vi "Configure IQ Output.vi"(0 "VISA resource name":refnum<visa-resource-name>, 1 "External Filter (1: Through)":u16(ring)=1 items=["40 MHz", "Through"], 2 "Enable Automatic External Filter (T:Enable)":bool=TRUE, 5 "Modulation Format (1: Dual Modulation)":u16(ring)=1 items=["Custom"=0, "Dual Modulation"=1, "Dual ARB"=2, "Multitone"=3, "Digital Modulation"=4, "Two-tone"=6, "AWGN Real-Time"=7, "AWGN ARB"=8], 7 "I/Q Attenuation Auto Mode (T:Enable)":bool=TRUE, 9 "I/Q Attenuation Level (2 dB)":dbl=2.0, 11 "error in (no error)":errorcluster, 12 "Enable Automatic Modulation Filter (T:Enable)":bool=TRUE, 13 "Modulation Filter (2: Through)":u16(ring)=2 items=["2.1 MHz", "40 MHz", "Through"]) -> (4 "VISA resource name out":refnum<visa-resource-name>, 15 "error out":errorcluster)   [LabVIEW 2018, in "Agilent PSG MXG Series.lvlib"]
doc: "Configures I/Q attenuation, external filter and modulation filter.\n\n<B>Notes:</B>\n(1) This VI is valid only in E8267C, E8257D, E8267D, N5162A, N5182A, N5172B, N5182B.\n\n(2) For E8267C, this VI is valid only when the instrument installs <B>Option 002</B> (Internal baseband generator) or <B>Option 602</B> (Digital bus baseband generator).\n\n(3) For E8267D, this VI is valid only when the instrument installs <B>Option 601</B> or <B>Option 602</B> (Internal baseband generator)."
uses:
  Agilent PSG MXG Series.lvlib
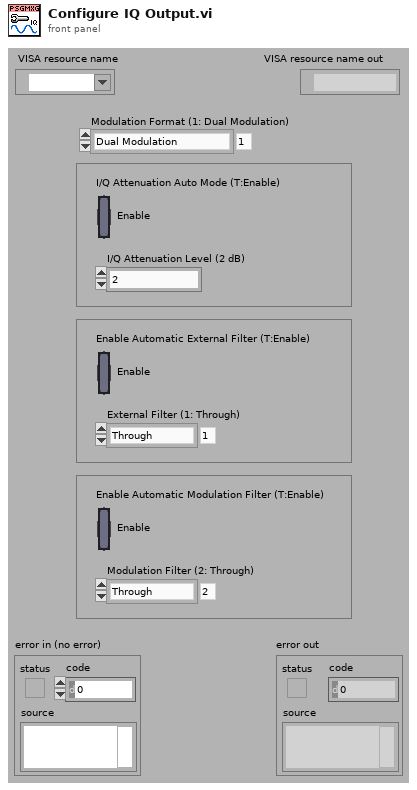
[diagram p1: front panel]
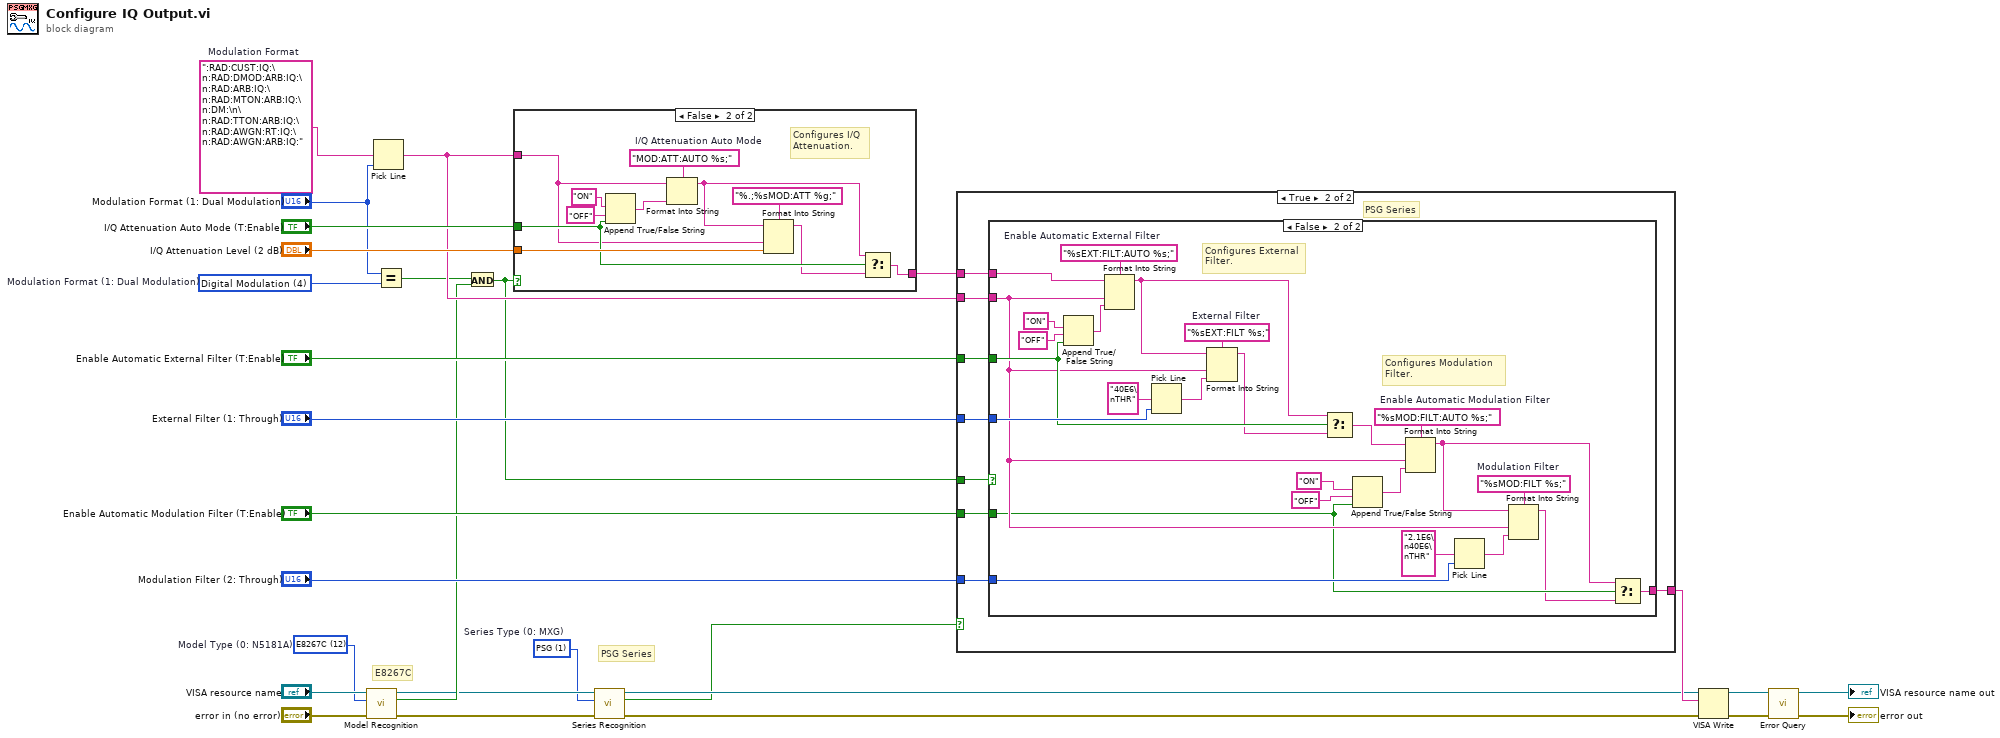
[diagram p0: block diagram]
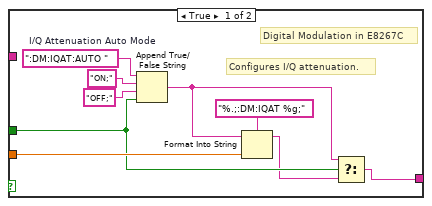
[diagram p2: hidden frame]
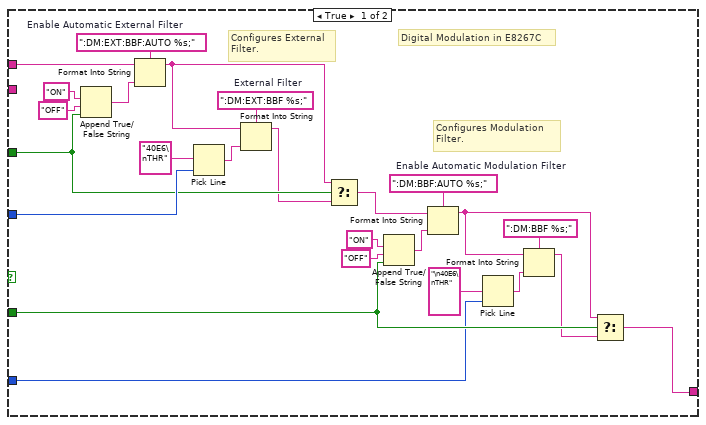
[diagram p4: hidden frame]
diagram:
  w5 = u16 4 items=["Custom"=0, "Dual Modulation"=1, "Dual ARB"=2, "Multitone"=3, "Digital Modulation"=4, "Two-tone"=6, "AWGN Real-Time"=7, "AWGN ARB"=8]  # Modulation Format (1: Dual Modulation)
  w6 = u16 1 items=["MXG-A", "PSG", "PSG-A", "PSG-C", "PSG-D", "MXG-B", "EXG"]  # Series Type (0: MXG)
  w7 = u16 12 items=["N5181A"=0, "N5182A"=1, "N5183A"=2, "N5161A"=3, "N5162A"=4, "E8241A"=5, "E8244A"=6, "E8251A"=7, "E8254A"=8, "E8247C"=10, "E8257C"=11, "E8267C"=12, "E8257D"=15, "E8267D"=16, "N5171B"=17, "N5172B"=18, "N5181B"=19, "N5182B"=20]  # Model Type (0: N5181A)
  w28 = ":RAD:CUST:IQ:\n:RAD:DMOD:ARB:IQ:\n:RAD:ARB:IQ:\n:RAD:MTON:ARB:IQ:\n:DM:\n\n:RAD:TTON:ARB:IQ:\n:RAD:AWGN:RT:IQ:\n:RAD:AWGN:ARB:IQ:"  # Modulation Format
  # "E8267C"
  # "PSG Series"
  n1 = call "Model Recognition.vi"("error in (no error)"="error in (no error)", "Model Type (0: N5181A)"=w7, "VISA resource name"="VISA resource name") -> ("error out"=w13:errorcluster, "Is Model Correct"=w15:bool, "VISA resource name out"=w14:refnum<visa-resource-name>)  [unwired: 6 out]
  n2 = Pick Line(multi-line string=w28, line index="Modulation Format (1: Dual Modulation)") -> (output string=w25:string)  [unwired: 1 out]
  n3 = Equal?(x="Modulation Format (1: Dual Modulation)", y=w5) -> (x = y?=w17:bool)
  n4 = And(x=w17, y=w15) -> (x .and. y?=w12:bool)
  n5 = case shown="False" w12 {
    tunnel: "I/Q Attenuation Level (2 dB)" -> [w34 w43]
    tunnel: "I/Q Attenuation Auto Mode (T:Enable)" -> [w32 w42]
    tunnel: w25 -> [_ w39]
    tunnel: [w29 w38] -> w24
    frame True {
      w37 = ":DM:IQAT:AUTO "  # I/Q Attenuation Auto Mode
      # "Configures I/Q attenuation."
      # "Digital Modulation in E8267C"
      n6 = Append True/False String(1:w32, 2:"OFF;" ("false string"), 3:"ON;" ("true string"), 4:w37) -> (0:w30:string)
      n7 = Format Into String(format string="%.;:DM:IQAT %g;", initial string=w30, w34) -> (resulting string=w31:string)  [unwired: 1 in, 1 out]
      n8 = Select(t=w30, s=w32, f=w31) -> (s? t:f=w29:string)
    }
    frame False {
      w48 = "MOD:ATT:AUTO %s;"  # I/Q Attenuation Auto Mode
      # "Configures I/Q\nAttenuation."
      n9 = Append True/False String(1:w42, 2:"OFF" ("false string"), 3:"ON" ("true string")) -> (0:w47:string)  [unwired: 1 out]
      n10 = Format Into String(format string=w48, initial string=w39, w47) -> (resulting string=w40:string)  [unwired: 1 in, 1 out]
      n11 = Format Into String(format string="%.;%sMOD:ATT %g;", initial string=w40, w39, w43) -> (resulting string=w41:string)  [unwired: 1 in, 1 out]
      n12 = Select(t=w40, s=w42, f=w41) -> (s? t:f=w38:string)
    }
  }
  n13 = call "Series Recognition.vi"("error in (no error)"=w13, "Series Type (0: MXG)"=w6, "VISA resource name"=w14) -> ("error out"=w2:errorcluster, "Is Series Correct"=w1:bool, "VISA resource name out"=w3:refnum<visa-resource-name>)  [unwired: 6 out]
  n14 = case shown="True" w1 {
    tunnel: w25 -> [_ w54]
    tunnel: w24 -> [w49 w57]
    tunnel: "Enable Automatic External Filter (T:Enable)" -> [_ w55]
    tunnel: "External Filter (1: Through)" -> [_ w56]
    tunnel: "Enable Automatic Modulation Filter (T:Enable)" -> [_ w52]
    tunnel: "Modulation Filter (2: Through)" -> [_ w53]
    tunnel: [w49 w51] -> w4
    tunnel: w12 -> [_ w50]
    frame False {
      # "MXG, EXG Series"
    }
    frame True {
      # "PSG Series"
      n15 = case shown="False" w50 {
        tunnel: w57 -> [w82 w107]
        tunnel: w56 -> [w74 w100]
        tunnel: w55 -> [w73 w99]
        tunnel: w54 -> [_ w90]
        tunnel: w53 -> [w61 w87]
        tunnel: w52 -> [w64 w86]
        tunnel: [w58 w83] -> w51
        frame True {
          w69 = ":DM:BBF:AUTO %s;"  # Enable Automatic Modulation Filter
          w77 = ":DM:EXT:BBF %s;"  # External Filter
          w81 = ":DM:EXT:BBF:AUTO %s;"  # Enable Automatic External Filter
          # "Configures Modulation\nFilter."
          # "Configures External\nFilter."
          # "Digital Modulation in E8267C"
          n16 = Append True/False String(1:w73, 2:"OFF" ("false string"), 3:"ON" ("true string")) -> (0:w80:string)  [unwired: 1 out]
          n17 = Format Into String(format string=w81, initial string=w82, w80) -> (resulting string=w71:string)  [unwired: 1 in, 1 out]
          n18 = Pick Line(multi-line string="40E6\nTHR", line index=w74) -> (output string=w76:string)  [unwired: 1 out]
          n19 = Format Into String(format string=w77, initial string=w71, w76) -> (resulting string=w72:string)  [unwired: 1 in, 1 out]
          n20 = Select(t=w71, s=w73, f=w72) -> (s? t:f=w70:string)
          n21 = Append True/False String(1:w64, 2:"OFF" ("false string"), 3:"ON" ("true string")) -> (0:w68:string)  [unwired: 1 out]
          n22 = Format Into String(format string=w69, initial string=w70, w68) -> (resulting string=w59:string)  [unwired: 1 in, 1 out]
          n23 = Pick Line(multi-line string="\n40E6\nTHR", line index=w61) -> (output string=w62:string)  [unwired: 1 out]
          n24 = Format Into String(format string=":DM:BBF %s;", initial string=w59, w62) -> (resulting string=w60:string)  [unwired: 1 in, 1 out]
          n25 = Select(t=w59, s=w64, f=w60) -> (s? t:f=w58:string)
        }
        frame False {
          w91 = "%sMOD:FILT %s;"  # Modulation Filter
          w95 = "%sMOD:FILT:AUTO %s;"  # Enable Automatic Modulation Filter
          w103 = "%sEXT:FILT %s;"  # External Filter
          w108 = "%sEXT:FILT:AUTO %s;"  # Enable Automatic External Filter
          # "Configures Modulation\nFilter."
          # "Configures External\nFilter."
          n26 = Append True/False String(1:w99, 2:"OFF" ("false string"), 3:"ON" ("true string")) -> (0:w104:string)  [unwired: 1 out]
          n27 = Format Into String(format string=w108, initial string=w107, w90, w104) -> (resulting string=w97:string)  [unwired: 1 in, 1 out]
          n28 = Pick Line(multi-line string="40E6\nTHR", line index=w100) -> (output string=w102:string)  [unwired: 1 out]
          n29 = Format Into String(format string=w103, initial string=w97, w90, w102) -> (resulting string=w98:string)  [unwired: 1 in, 1 out]
          n30 = Select(t=w97, s=w99, f=w98) -> (s? t:f=w96:string)
          n31 = Append True/False String(1:w86, 2:"OFF" ("false string"), 3:"ON" ("true string")) -> (0:w94:string)  [unwired: 1 out]
          n32 = Format Into String(format string=w95, initial string=w96, w90, w94) -> (resulting string=w84:string)  [unwired: 1 in, 1 out]
          n33 = Pick Line(multi-line string="2.1E6\n40E6\nTHR", line index=w87) -> (output string=w89:string)  [unwired: 1 out]
          n34 = Format Into String(format string=w91, initial string=w84, w90, w89) -> (resulting string=w85:string)  [unwired: 1 in, 1 out]
          n35 = Select(t=w84, s=w86, f=w85) -> (s? t:f=w83:string)
        }
      }
    }
  }
  n36 = VISA Write(VISA resource name=w3, write buffer=w4, error in (no error)=w2) -> (VISA resource name out=w19:refnum<visa-resource-name>, error out=w18:errorcluster)  [unwired: 1 out]
  n37 = call "Error Query.vi"("error in (no error)"=w18, "VISA resource name"=w19) -> ("error out"=→"error out":errorcluster, "VISA resource name out"=→"VISA resource name out":refnum<visa-resource-name>)  [unwired: 8 out]
